vi "Request Addresses.vi"(8 "error in (no error)":errorcluster, 11 "connection info":T2) -> (0 "error out":errorcluster, 2 "All Data":T1[](array[typedef]) {"Name" format="%.0x"}, 3 "connection info":T2)   [LabVIEW 2015, in "J1939 Addon Shared.lvlib"]
uses:
  J1939 Addon Shared.lvlib
  <vilib>/NI/STM/TCP/TCP Connection Info.ctl
  <vilib>/NI/STM/SubVIs/MetaDataElement.ctl
  Types/Address Lookup Table Data.ctl
  <vilib>/NI/NIVS Addon Network Comm/Shared/NI VeriStand Addon Network Comm Shared.lvlib
  <vilib>/NI/STM/NI STM.lvlib
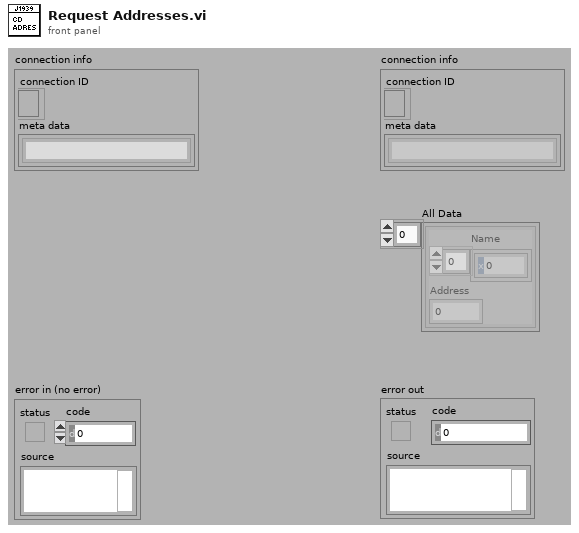
[diagram p1: front panel]
types:
  T1 = typedef "J1939 Addon Shared.lvlib/Address Lookup Table Data.ctl" = cluster{"Name":u8[], "Address":u8}
  T2 = typedef "NI STM.lvlib/TCP Connection Info.ctl" = cluster{"connection ID":refnum<k5>, "meta data":T3[]}
  T3 = typedef "NI STM.lvlib/MetaDataElement.ctl" = string
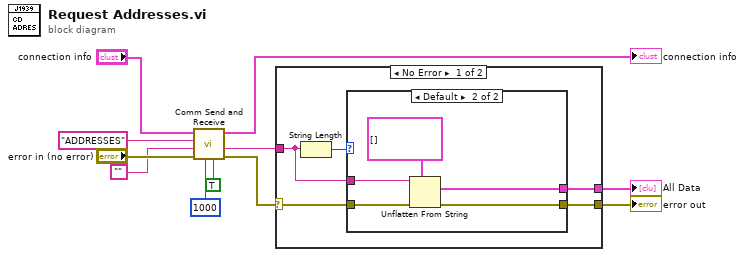
[diagram p0: block diagram]
diagram:
  n1 = call <vilib>:"Comm Send and Receive.vi"("Resp Required?"=TRUE, "Timeout (ms)"=u32 1000 ("Timeout ms (5000)"), "error in (no error)"="error in (no error)", "Data"="", "Name"="ADDRESSES" ("Command"), "connection info"="connection info") -> ("error out"=w6:errorcluster, "Data"=w3:string, "connection info"=→"connection info":T2)  [unwired: 2 in, 1 out]
  n2 = case shown="No Error" w6 {
    selector: w6 -> [w15 w23]
    tunnel: w3 -> [w12 _]
    tunnel: [w14 w23] -> w10
    tunnel: [w13 _] -> w11
    frame No Error {
      n3 = String Length(string=w12) -> (length=w16:i32)
      n4 = case shown="Default" w16 {
        tunnel: w15 -> [w17 w21]
        tunnel: w12 -> [_ w20]
        tunnel: [w17 w19] -> w14
        tunnel: [_ w18] -> w13
        frame 0 {
        }
        frame Default {
          n5 = Unflatten From String(type=T1[] [] ("All Data"), binary string=w20, error in (no error)=w21) -> (value=w18:T1[], error out=w19:errorcluster)  [unwired: 2 in, 1 out]
        }
      }
    }
    frame Error {
    }
  }
  "All Data" <- w11
  "error out" <- w10
